vi "StringVariableParse.vi"(8 "error in":errorcluster, 9 "Info":T1, 10 "in":string, 11 "dictionary":T2) -> (0 "error out":errorcluster, 2 "out":string, 3 "Find?":bool)   [LabVIEW 2018]
uses:
  <userlib>/_OpenG.lib/dictionary/dictionary.llb/Dictionary Object RefNum__ogtk.ctl
  <userlib>/_OpenG.lib/dictionary/dictionary.llb/Dictionary Object RefNum - Enum__ogtk.ctl
  <vilib>/regexp/Match Regular Expression.xnode
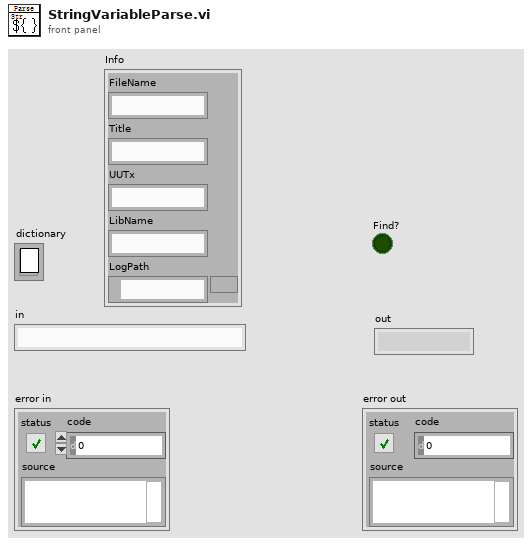
[diagram p1: front panel]
types:
  T1 = cluster{"FileName":string, "Title":string, "UUTx":string, "LibName":string, "LogPath":path}
  T2 = typedef "Dictionary Object RefNum__ogtk.ctl" = refnum<k1>
  T3 = cluster{"Describe":string, "ValueArray":string[]}
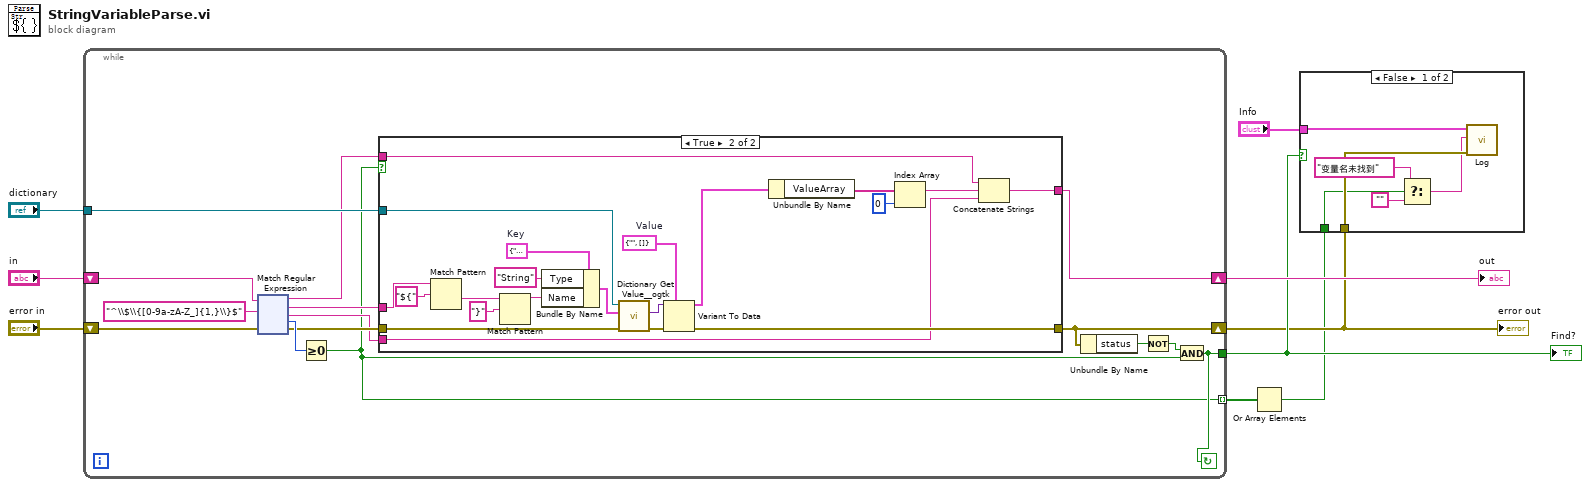
[diagram p0: block diagram]
diagram:
  n1 = while {
    tunnel: "dictionary" -> [w23]
    tunnel: [w11] -> w5
    shift-right: [w21] -> w3
    shift-left: "error in" -> [w22]
    shift-right: [w12] -> w6
    shift-left: "in" -> [w24]
    tunnel: [w10] -> w2 mode=indexing
    stop <- w11 continue-if-true
    n2 = xnode "Match Regular Expression"("input string"=w24, "regular expression"="^\\$\\{[0-9a-zA-Z_]{1,}\\}$", "error in"=w22) -> ("before match"=w14:string, "whole match"=w18:string, "after match"=w13:string, "offset past match"=w19:i32, "error out"=w15:errorcluster)  [unwired: 3 in]
    n3 = Greater Or Equal To 0?(x=w19) -> (x >= 0?=w10:bool)
    n4 = case shown="True" w10 {
      tunnel: [w25 w29] -> w12
      tunnel: w23 -> [_ w45]
      tunnel: w18 -> [_ w41]
      tunnel: w15 -> [w26 w40]
      tunnel: [w26 w39] -> w21
      tunnel: w14 -> [w25 w28]
      tunnel: w13 -> [_ w27]
      frame False {
      }
      frame True {
        w35 = T3 {"Describe"="", "ValueArray"=[]}  # Value
        w38 = cluster{"Type":string, "Name":string} {"Type"="", "Name"=""}  # Key
        n5 = Match Pattern(string=w41, regular expression="${") -> (after substring=w44:string)  [unwired: 1 in, 3 out]
        n6 = Match Pattern(string=w44, regular expression="}") -> (before substring=w37:string)  [unwired: 1 in, 3 out]
        n7 = Bundle By Name(cluster=w38, "Type"="String", "Name"=w37) -> (w36:cluster{"Type":string, "Name":string})
        n8 = call <userlib>:"Dictionary Get Value__ogtk.vi"("error in"=w40, "key"=w36, "dictionary"=w45) -> ("error out"=w47:errorcluster, "value"=w46:variant)  [unwired: 5 in, 2 out]
        n9 = Variant To Data(error in=w47, type=w35, Variant=w46) -> (data=w34:T3, error out=w39:errorcluster)
        n10 = Unbundle By Name(w34) -> ("ValueArray"=w33:string[])
        n11 = Index Array(array=w33, index=0) -> (element=w31:string)
        n12 = Concatenate Strings(w28, w31, w27) -> (w29:string)
      }
    }
    n13 = Unbundle By Name(w21) -> ("status"=w17:bool)
    n14 = Not(x=w17) -> (.not. x?=w16:bool)
    n15 = And(x=w16, y=w10) -> (x .and. y?=w11:bool)
  }
  "error out" <- w3
  "Find?" <- w5
  "out" <- w6
  n16 = Or Array Elements(Boolean array=w2) -> (logical OR=w1:bool)
  n17 = case shown="False" w5 {
    tunnel: "Info" -> [w167 _]
    tunnel: w3 -> [w166 _]
    tunnel: w1 -> [w165 _]
    frame False {
      n18 = Select(t="变量名未找到" ("LogIn"), s=w165, f="") -> (s? t:f=w163:string)
      n19 = call "Log.vi"("error in"=w166, "LogIn"=w163, "Info"=w167) -> ()  [unwired: 9 in]
    }
    frame True {
    }
  }
